vi "Init.vi"(8 "error in (no error)":errorcluster, 10 "Slot Name":string, 11 "Data Realm":T1) -> (0 "error out":errorcluster, 3 "GetPersistentData out":refnum<class "GetPersistentData.lvclass">)   [LabVIEW 2020, in "obs-websocket.lvlib" / "GetPersistentData.lvclass"]
uses:
  GetPersistentData.lvclass
  Data Realm.ctl
  obs-websocket.lvlib
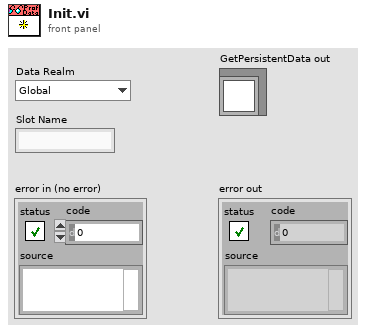
[diagram p1: front panel]
types:
  T1 = typedef "obs-websocket.lvlib/Data Realm.ctl" = enum16{"Global", "Profile"}
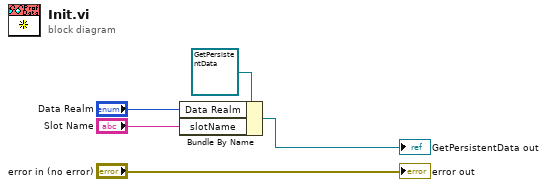
[diagram p0: block diagram]
diagram:
  n1 = Bundle By Name(cluster=refnum<class "GetPersistentData.lvclass"> refnum ("GetPersistentData in"), "Data Realm"="Data Realm", "slotName"="Slot Name") -> (→"GetPersistentData out":refnum<class "GetPersistentData.lvclass">)
  "error out" <- "error in (no error)"
